vi "Create Template Config File.vi"(11 "configuration file path":path=path "/home/lvuser/example.ini") -> (0 "error out":errorcluster)   [LabVIEW 2014]
uses:
  <vilib>/Utility/config.llb/Write Key (String).vi
  Lidar Distance Global.vi
  Begin Cals.vi
  DriveTrainCals.vi
  AutonCals.vi
  <vilib>/Utility/config.llb/NI_LVConfig.lvlib
panel:
  out "DriveP":dbl=1.0
  out "MinUltraSonic":dbl=10.0
  out "Encoder Distance Per Rotation":dbl
  out "Lidar_Distance":dbl
  in  "OK Button":bool
  out "IgnoreErrors":errorcluster
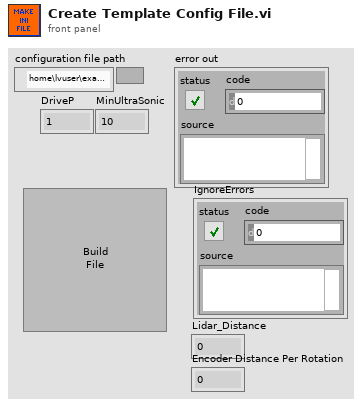
[diagram p1: front panel]
types:
  T1 = typedef "NI_LVConfig.lvlib/Config Data RefNum.ctl" = refnum<k1>
  T2 = enum32{"invalid VI type", "Standard VI", "Control VI", "Global VI", "Polymorphic VI", "Configuration VI", "SubSystem", "Facade VI", "Method VI", "Statechart Diagram VI"}
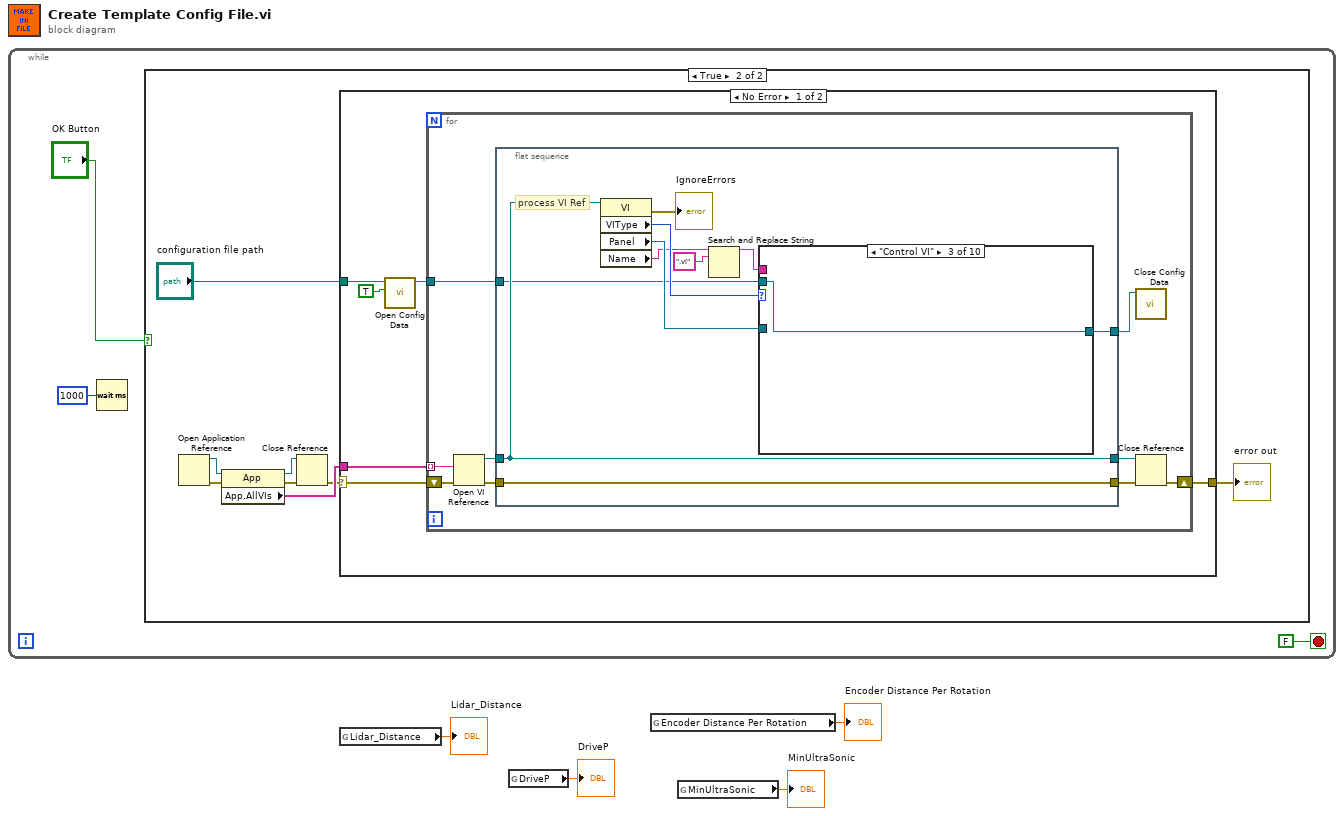
[diagram p0: block diagram]
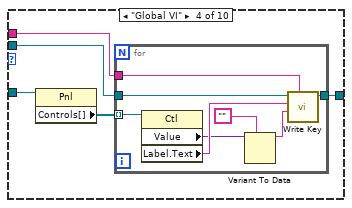
[diagram p5: hidden frame]
diagram:
  n1 = while {
    stop <- FALSE stop-if-true
    n2 = Wait (ms)(milliseconds to wait=u32 1000) -> ()  [unwired: 1 out]
    n3 = case shown="True" "OK Button" {
      frame False {
      }
      frame True {
        n4 = Open Application Reference() -> (0:w11:errorcluster, 3:w8:refnum<vi>)  [unwired: 4 in]
        n5 = property class="App"(reference=w8, error in=w11) -> (reference out=w9:refnum<vi>, error out=w10:errorcluster, "App.AllVIs"=w13:string[])
        n6 = Close Reference(reference=w9, error in (no error)=w10) -> (error out=w12:errorcluster)
        n7 = case shown="No Error" w12 {
          selector: w12 -> [w20 w63]
          tunnel: w13 -> [w21 _]
          tunnel: [w19 w63] -> w14
          tunnel: "configuration file path" -> [w17 _]
          frame No Error {
            n8 = call <vilib>:"Open Config Data.vi"("create file if necessary (T)"=TRUE, "configuration file path"=w17) -> ("refnum"=w18:T1)  [unwired: 7 in, 2 out]
            n9 = for {
              tunnel: w21 -> [w30] mode=indexing
              shift-right: [w24] -> w19
              shift-left: w20 -> [w25]
              tunnel: w18 -> [w23]
              n10 = Open VI Reference(vi path=w30, error in (no error)=w25) -> (vi reference=w29:refnum<vi>, error out=w27:errorcluster)  [unwired: 4 in]
              n11 = flat-sequence {
                tunnel: w29 -> [w39]
                tunnel: [w39] -> w28
                tunnel: w27 -> [w40]
                tunnel: [w40] -> w26
                tunnel: w23 -> [w33]
                tunnel: [w31] -> w22
                frame #0 {
                  # "process VI Ref"
                  n12 = property class="VI"(reference=w39) -> (error out=→"IgnoreErrors":errorcluster, "VIType"=w38:T2, "Panel"=w37:refnum<vi>, "Name"=w36:string)  [unwired: 1 in, 1 out]
                  n13 = Search and Replace String(input string=w36, search string=".vi" ("substring (\"\")")) -> (result string=w34:string)  [unwired: 6 in, 3 out]
                  n14 = case shown="\"Control VI\"" w38 {
                    tunnel: w37 -> [_ _ _ w48 _ _ _ _ _ _]
                    tunnel: w34 -> [_ _ _ w45 _ _ _ _ _ _]
                    tunnel: w33 -> [w41 w42 w43 w46 w57 w58 w59 w60 w61 w62]
                    tunnel: [w41 w42 w43 w44 w57 w58 w59 w60 w61 w62] -> w31
                    frame "invalid VI type", Default {
                    }
                    frame "Standard VI" {
                    }
                    frame "Control VI" {
                    }
                    frame "Global VI" {
                      n15 = property class="Pnl"(reference=w48) -> ("Controls[]"=w47:refnum<vi>[])  [unwired: 1 in, 2 out]
                      n16 = for {
                        tunnel: w47 -> [w56] mode=indexing
                        tunnel: w46 -> [w55]
                        tunnel: w45 -> [w54]
                        tunnel: [w49] -> w44
                        n17 = property class="Ctl"(reference=w56) -> ("Value"=w52:variant, "Label.Text"=w53:string)  [unwired: 1 in, 2 out]
                        n18 = Variant To Data(type="", Variant=w52) -> (data=w50:string)  [unwired: 1 in, 1 out]
                        n19 = call-poly <vilib>:"Write Key.vi"("section"=w54, "value"=w50, "key"=w53, "refnum"=w55) -> ("refnum out"=w49:T1)  [unwired: 5 in, 2 out]
                      }
                    }
                    frame "Polymorphic VI" {
                    }
                    frame "Configuration VI" {
                    }
                    frame "SubSystem" {
                    }
                    frame "Facade VI" {
                    }
                    frame "Method VI" {
                    }
                    frame "Statechart Diagram VI" {
                    }
                  }
                }
              }
              n20 = call <vilib>:"Close Config Data.vi"("refnum"=w22) -> ()  [unwired: 9 in, 2 out]
              n21 = Close Reference(reference=w28, error in (no error)=w26) -> (error out=w24:errorcluster)
            }
          }
          frame Error {
          }
        }
        "error out" <- w14
      }
    }
  }
  n22 = global read "Lidar Distance Global.vi" "Lidar_Distance"() -> (→"Lidar_Distance":dbl)
  n23 = global read "AutonCals.vi" "DriveP"() -> (→"DriveP":dbl)
  n24 = global read "Begin Cals.vi" "Encoder Distance Per Rotation"() -> (→"Encoder Distance Per Rotation":dbl)
  n25 = global read "DriveTrainCals.vi" "MinUltraSonic"() -> (→"MinUltraSonic":dbl)
